vi "get Retract wfm.vi"(0 "reference in":refnum<class "Fcurve.lvclass">, 1 "Zeroed (wfms.array)":waveform(dbl)[](array[waveform]), 2 "End contact (index)":i32, 5 "error in (no error)":errorcluster) -> (14 "reference out":refnum<class "Fcurve.lvclass">, 15 "Zeroed (wfms.array) out":waveform(dbl)[](array[waveform]), 16 "Samples retract out":i32, 17 "Retract indices [start,end]":cluster{"Start":i32, "End":i32}, 18 "Retract":cluster{"X":dbl[], "Y":dbl[]}, 19 "error out":errorcluster)   [LabVIEW 2019, in "Fcurve.lvclass"]
uses:
  Fcurve.lvclass
  Fcurve sections.ctl
  <vilib>/Waveform/WDTOps.llb/WDT Get Waveform Subset DBL.vi
panel:
  out "x-y":i32
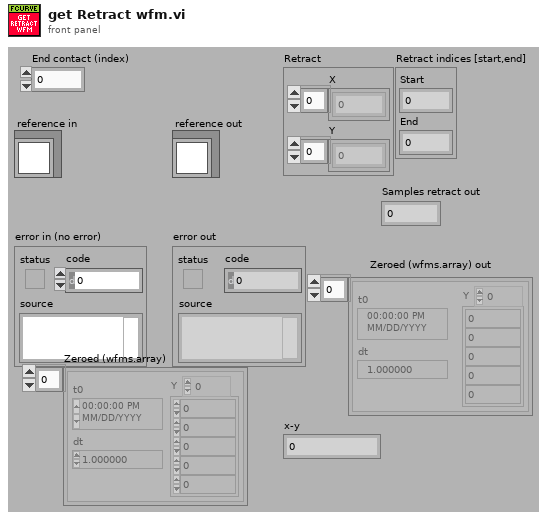
[diagram p1: front panel]
types:
  T1 = typedef "Fcurve.lvclass/Fcurve sections.ctl" = enum16{"Approach", "Contact", "Retract"}
  T2 = typedef "Fcurve.lvclass/ObjectAttributes.ctl" = cluster{"MyAttribute":dbl, "Fcurve Metadata":T3, "Contact Spread of dev":dbl, "Tau Delay (ms)":dbl, "Points of contact":dbl, "Def_wfm":cluster{"Max":dbl, "Min":dbl}, "Zpos_wfm":cluster{"Max":dbl, "Min":dbl}, "Contact stat?":bool, "Real AI dt (s)":dbl, "Decimation":cluster{"App":cluster{"Dec":i32, "apply":bool}, "Con":cluster{"Dec":i32, "apply":bool}, "Ret":cluster{"Dec":i32, "apply":bool}}, "Segment def[0]":dbl, "Segment Zpos[0]":dbl, "Raw Datum":waveform(dbl)[], "Group metadata":T4, "M_data obj":refnum<class "metadata.lvclass">, "Channel name(s)":string[], "Segment fcurve data":cluster{"X":dbl[], "Y":dbl[]}[], "Segment duration":cluster{"Start":i32, "Duration":i32}[], "Segment info":T5[], "Segment durations (S)":dbl[], "Segments Maxmin":T7[]}
  T3 = typedef "Fcurve.lvclass/Metadata.ctl" = cluster{"dt (us)":dbl, "Dec Factor":dbl, "Z piezo Sensitivity (nm/V)":dbl, "K (N/m)":dbl, "Sp (V)":dbl, "Contact (ms)":dbl, "Zpos contact":dbl, "Vel_app (nm/s)":dbl, "Vel_ret (nm/s)":dbl, "deltaV (nm)":dbl, "Def_V0 (v)":dbl, "Piezo gain":dbl, "invOLS (nm/V)":dbl}
  T4 = typedef "TDMS_DataHandler.lvclass/Fcurve Meta data.ctl" = cluster{"property names":string[], "property values":variant[]}
  T5 = typedef "Fcurve.lvclass/Fcurve segments --cluster.ctl" = cluster{"type":T6, "nb points":i32, "dec factor":u32, "sampling rate (S/s)":u32}
  T6 = typedef "metadata.lvclass/Segment type--combobox.ctl" = string
  T7 = typedef "Fcurve.lvclass/Segment MaxMin --cluster.ctl" = cluster{"Def":cluster{"max value":dbl, "min value":dbl}, "Zpos":cluster{"max value":dbl, "min value":dbl}}
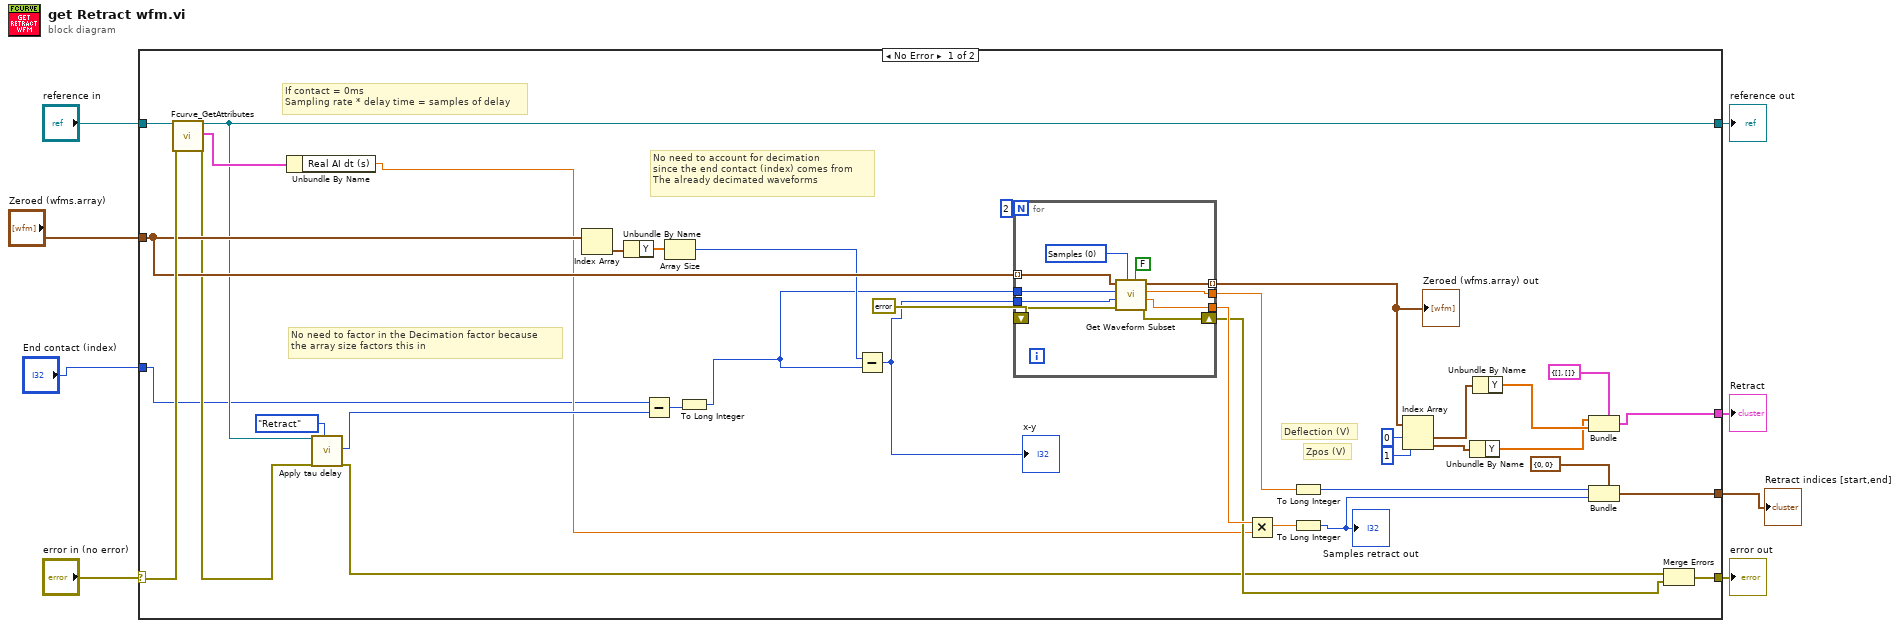
[diagram p0: block diagram]
diagram:
  n1 = case shown="No Error" "error in (no error)" {
    selector: "error in (no error)" -> [w44 w57]
    tunnel: [w45 w57] -> w7
    tunnel: [w17 w56] -> w5
    tunnel: "reference in" -> [w41 w56]
    tunnel: [w24 _] -> w4
    tunnel: [w23 _] -> w3
    tunnel: "End contact (index)" -> [w11 _]
    tunnel: "Zeroed (wfms.array)" -> [w22 _]
    frame No Error {
      # "No need to account for decimation\nsince the end contact (index) comes from\nThe already decimated waveforms"
      # "No need to factor in the Decimation factor because\nthe array size factors this in"
      # "Deflection (V)"
      # "Zpos (V)"
      # "If contact = 0ms\nSampling rate * delay time = samples of delay"
      n2 = call "Fcurve_GetAttributes.vi"("reference in"=w41, "error in (no error)"=w44) -> ("reference out"=w17:refnum<class "Fcurve.lvclass">, "attributes"=w43:T2, "error out"=w16:errorcluster)  [unwired: 14 in, 1 out]
      n3 = Unbundle By Name(w43) -> ("Real AI dt (s)"=w12:dbl)
      n4 = call "Apply tau delay.vi"("reference in"=w17, "error in (no error)"=w16, "Section"=Fcurve_sections."Retract") -> ("# of samples"=w15:i32, "error out"=w10:errorcluster)  [unwired: 13 in, 2 out]
      n5 = Index Array(array=w22) -> (element=w34:waveform(dbl))  [unwired: 1 in]
      n6 = Unbundle By Name(w34) -> ("Y"=w33:dbl[])
      n7 = Subtract(x=w11, y=w15) -> (x-y=w14:i32)
      n8 = Array Size(array=w33) -> (size(s)=w19:i32)
      n9 = To Long Integer(number=w14) -> (32bit integer=w13:i32)
      n10 = Subtract(x=w19, y=w13) -> (x-y=w18:i32)
      "x-y" <- w18
      n11 = for {
        N: 2 -> [_]
        tunnel: [w54] -> w42
        tunnel: [w53] -> w39 mode=indexing
        tunnel: w22 -> [w52] mode=indexing
        shift-right: [w49] -> w25
        shift-left: errorcluster {"status"=FALSE, "code"=0, "source"=""} ("error out") -> [w50]
        tunnel: [w48] -> w30
        tunnel: w13 -> [w47]
        tunnel: w18 -> [w46]
        w55 = u16 0 items=["Samples", "Relative Time"] ("start/duration format")
        n12 = call-poly <vilib>:"Get Waveform Subset.vi"("open interval? (T)"=FALSE, "start/duration format"=w55, "error in (no error)"=w50, "duration"=w46, "start samples/time"=w47, "waveform in"=w52) -> ("error out"=w49:errorcluster, "actual duration"=w54:dbl, "actual start samples/time"=w48:dbl, "waveform out"=w53:waveform(dbl))
      }
      "Zeroed (wfms.array) out" <- w39
      n13 = Multiply(x=w42, y=w12) -> (x*y=w35:dbl)
      n14 = To Long Integer(number=w30) -> (32bit integer=w29:i32)
      n15 = To Long Integer(number=w35) -> (32bit integer=w31:i32)
      "Samples retract out" <- w31
      n16 = Index Array(array=w39, index #1=0 ("index"), index #2=1 ("index")) -> (element #1=w38:waveform(dbl), element #2=w37:waveform(dbl))
      n17 = Unbundle By Name(w37) -> ("Y"=w20:dbl[])
      n18 = Unbundle By Name(w38) -> ("Y"=w21:dbl[])
      n19 = Bundle(cluster=cluster{"X":dbl[], "Y":dbl[]} {"X"=[], "Y"=[]} ("Fcurve.Approach"), "X"=w20, "Y"=w21) -> (w24:cluster{"X":dbl[], "Y":dbl[]})
      n20 = Bundle(cluster=cluster{"Start":i32, "End":i32} {"Start"=0, "End"=0} ("Fcurve index.Retract indices"), "Start"=w29, "End"=w31) -> (w23:cluster{"Start":i32, "End":i32})
      n21 = Merge Errors(w10, w25) -> (w45:errorcluster)
    }
    frame Error {
    }
  }
  "error out" <- w7
  "reference out" <- w5
  "Retract" <- w4
  "Retract indices [start,end]" <- w3
